vi "Timer.vi"(8 "error in (no error)":errorcluster, 11 "Attributes in":refnum<class "Attributes.lvclass">) -> (0 "error out":errorcluster, 2 "Complete?":bool, 3 "Attributes out":refnum<class "Attributes.lvclass">)   [LabVIEW 2021, in "Attributes.lvclass"]
uses:
  Attributes.lvclass
  Attributes.lvclass/Attributes.ctl
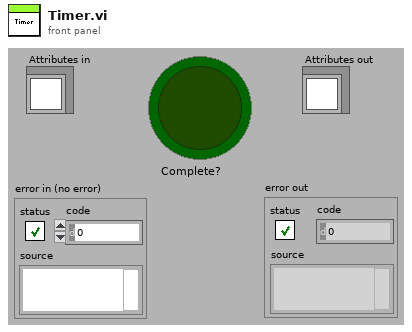
[diagram p1: front panel]
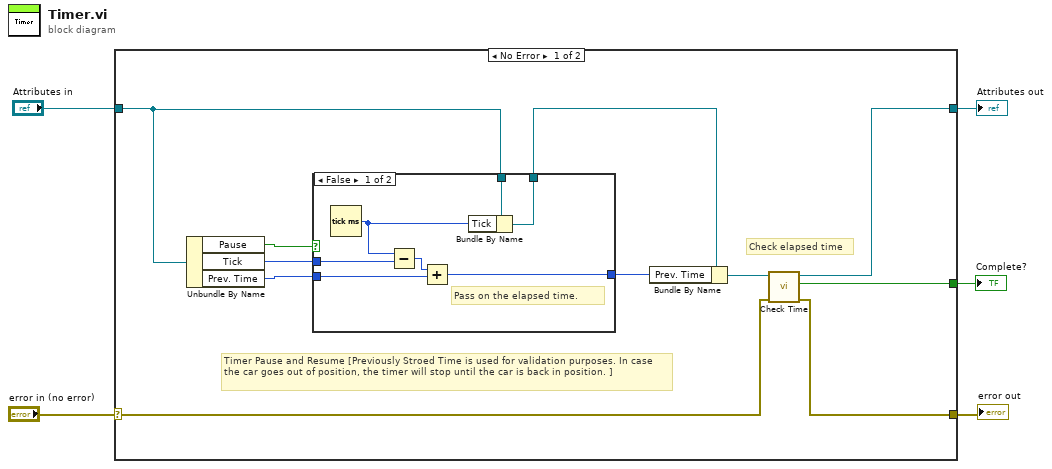
[diagram p0: block diagram]
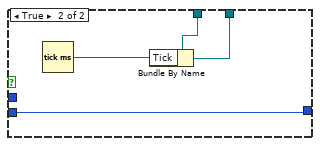
[diagram p2: hidden frame]
diagram:
  n1 = case shown="No Error" "error in (no error)" {
    selector: "error in (no error)" -> [w12 w29]
    tunnel: [w11 w29] -> w4
    tunnel: [w9 w28] -> w2
    tunnel: "Attributes in" -> [w7 w28]
    tunnel: [w8 _] -> w1
    frame No Error {
      # "Check elapsed time"
      # "Timer Pause and Resume [Previously Stroed Time is used for validation purposes. In case the car goes out of position, the timer will stop until the car is back in position. ]"
      n2 = Unbundle By Name(w7) -> ("Pause"=w16:bool, "Tick"=w15:u32, "Prev. Time"=w14:u32)
      n3 = case shown="False" w16 {
        tunnel: w15 -> [w23 _]
        tunnel: w14 -> [w21 w27]
        tunnel: [w20 w27] -> w13
        tunnel: w7 -> [w19 w25]
        tunnel: [w18 w24] -> w6
        frame False {
          # "Pass on the elapsed time."
          n4 = Tick Count (ms)() -> (millisecond timer value=w17:u32)
          n5 = Subtract(x=w17, y=w23) -> (x-y=w22:u32)
          n6 = Add(x=w22, y=w21) -> (x+y=w20:u32)
          n7 = Bundle By Name(cluster=w19, "Tick"=w17) -> (w18:refnum<class "Attributes.lvclass">)
        }
        frame True {
          n8 = Tick Count (ms)() -> (millisecond timer value=w26:u32)
          n9 = Bundle By Name(cluster=w25, "Tick"=w26) -> (w24:refnum<class "Attributes.lvclass">)
        }
      }
      n10 = Bundle By Name(cluster=w6, "Prev. Time"=w13) -> (w10:refnum<class "Attributes.lvclass">)
      n11 = call-dynamic "Check Time.vi"("error in (no error)"=w12, "Attributes in"=w10) -> ("error out"=w11:errorcluster, "Complete?"=w8:bool, "Attributes out"=w9:refnum<class "Attributes.lvclass">)  [unwired: 7 in]
    }
    frame Error {
      # "If there's an error pass on the attributes unchanged."
    }
  }
  "error out" <- w4
  "Attributes out" <- w2
  "Complete?" <- w1
